vi "TCP Client.vi"() -> ()   [LabVIEW 2014]
panel:
  in  "정지":bool
  out "웨이브폼 그래프":dbl[](graph)
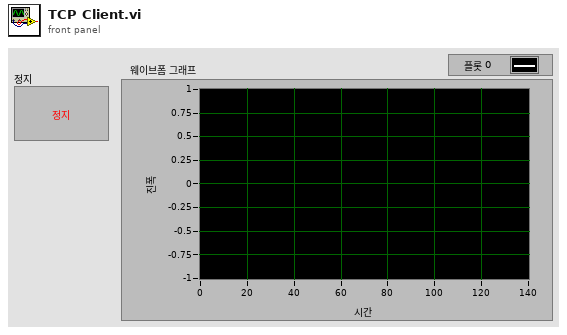
[diagram p1: front panel]
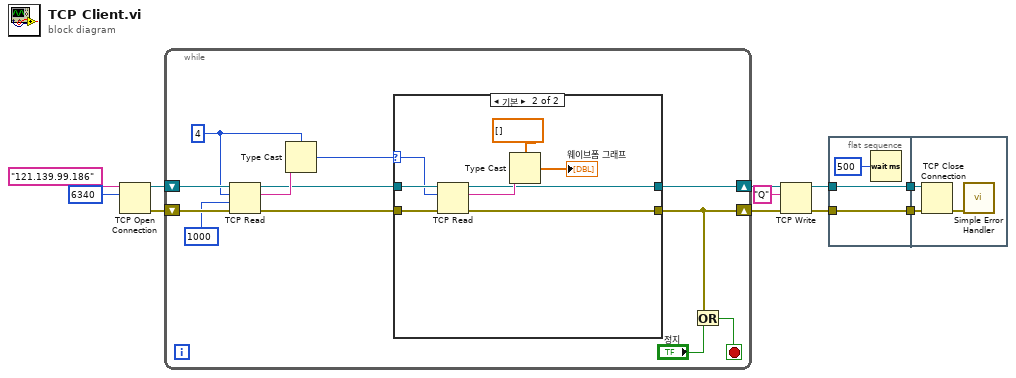
[diagram p0: block diagram]
diagram:
  n1 = TCP Open Connection(address="121.139.99.186" ("주소"), remote port or service name=u16 6340 ("원격 포트 또는 서비스 이름")) -> (connection ID=w9:refnum<k5>, error out=w8:errorcluster)  [unwired: 3 in]
  n2 = while {
    shift-right: [w17] -> w6
    shift-left: w9 -> [w23]
    shift-right: [w13] -> w7
    shift-left: w8 -> [w22]
    stop <- w14 stop-if-true
    w19 = 4 ("읽을 바이트")
    n3 = TCP Read(connection ID=w23, bytes to read=w19, error in (no error)=w22, 9:1000 ("읽을 바이트")) -> (connection ID out=w18:refnum<k5>, data out=w20:string, error out=w16:errorcluster)  [unwired: 1 in]
    n4 = Type Cast(type=w19, x=w20) -> (*(type *) &x=w15:i32)
    n5 = case shown="기본" w15 {
      selector: w15 -> [_ w31]
      tunnel: w18 -> [w25 w33]
      tunnel: [w25 w28] -> w17
      tunnel: w16 -> [w24 w32]
      tunnel: [w24 w27] -> w13
      frame 0 {
      }
      frame Default {
        n6 = TCP Read(connection ID=w33, bytes to read=w31, error in (no error)=w32) -> (connection ID out=w28:refnum<k5>, data out=w29:string, error out=w27:errorcluster)  [unwired: 2 in]
        n7 = Type Cast(type=dbl[] [], x=w29) -> (*(type *) &x=→"웨이브폼 그래프":dbl[])
      }
    }
    n8 = Or(x=w13, y="정지") -> (x .or. y?=w14:bool)
  }
  n9 = TCP Write(connection ID=w6, data in="Q" ("데이터 입력"), error in (no error)=w7) -> (connection ID out=w3:refnum<k5>, error out=w4:errorcluster)  [unwired: 1 in, 1 out]
  n10 = flat-sequence {
    tunnel: w3 -> [w35]
    tunnel: w4 -> [w36]
    tunnel: [w36] -> w2
    tunnel: [w35] -> w1
    tunnel: w2 -> [w39]
    tunnel: w1 -> [w38]
    frame #0 {
      n11 = Wait (ms)(milliseconds to wait=u32 500 ("대기 시간(ms)")) -> ()  [unwired: 1 out]
    }
    frame #1 {
      n12 = TCP Close Connection(connection ID=w38, error in (no error)=w39) -> (error out=w37:errorcluster)  [unwired: 1 in, 1 out]
      n13 = call <vilib>:"Simple Error Handler.vi"("error in (no error)"=w37) -> ()  [unwired: 4 in, 5 out]
    }
  }
